vi "ApplyLayoutToObject.vi"(5 "scaling settings":T1={"scaling factor"={"horizontal"=1.0, "vertical"=1.0}, "scale text"=FALSE} {"scaling factor"."vertical" min=0.0; "scaling factor"."horizontal" min=0.0}, 7 "properties to ignore":variant, 8 "error in (no error)":errorcluster, 10 "GObj Refnum":refnum<vi>, 11 "Object Layout in":refnum<class "Object Layout.lvclass">) -> (0 "error out":errorcluster, 3 "Object Layout out":refnum<class "Object Layout.lvclass">)   [LabVIEW 2012, in "NI_SE_Front Panel Layout.lvlib" / "Object Layout.lvclass"]
doc: "Apply layout information to the GObj Refnum."
uses:
  Object Layout.lvclass
  Scaling Factor_Options.ctl
  XY Scaling Factor.ctl
  Object Layout.lvclass/Object Layout.ctl
  Properties To Ignore.vi
  Set FP Object Size.vi
  NI_SE_Front Panel Layout.lvlib
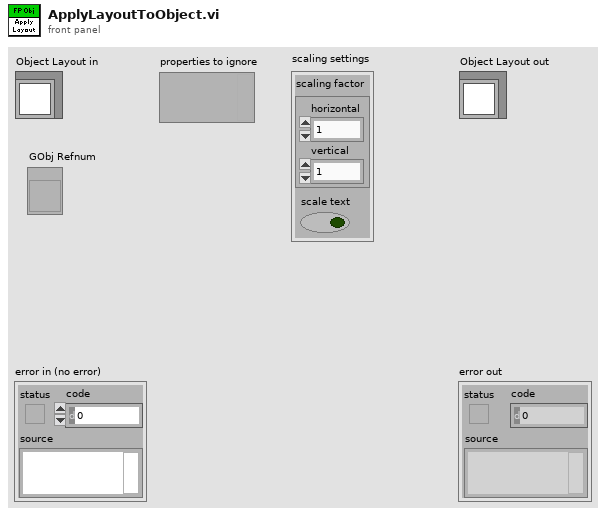
[diagram p1: front panel]
types:
  T1 = typedef "NI_SE_Front Panel Layout.lvlib/Scaling Factor_Options.ctl" = cluster{"scaling factor":T2, "scale text":bool}
  T2 = typedef "NI_SE_Front Panel Layout.lvlib/XY Scaling Factor.ctl" = cluster{"horizontal":dbl, "vertical":dbl}
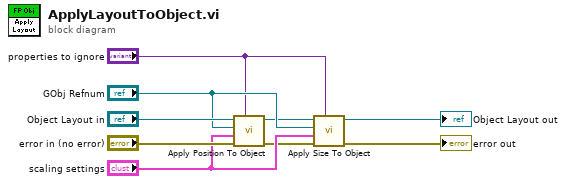
[diagram p0: block diagram]
diagram:
  n1 = call "Apply Position To Object.vi"("properties to ignore"="properties to ignore", "error in (no error)"="error in (no error)", "scaling settings"="scaling settings", "GObj Refnum"="GObj Refnum", "NI_SE_Object Layout in"="Object Layout in") -> ("error out"=w2:errorcluster, "NI_SE_Object Layout out"=w1:refnum<class "Object Layout.lvclass">)  [unwired: 5 in]
  n2 = call "Apply Size To Object.vi"("properties to ignore"="properties to ignore", "error in (no error)"=w2, "scaling settings"="scaling settings", "GObj Refnum"="GObj Refnum", "NI_SE_Object Layout in"=w1) -> ("error out"=→"error out":errorcluster, "NI_SE_Object Layout out"=→"Object Layout out":refnum<class "Object Layout.lvclass">)  [unwired: 5 in]
